vi "参数设置对话框.vi"() -> ()   [LabVIEW 2016, in "科盛超标留样.lvlib"]
uses:
  <vilib>/Utility/config.llb/NI_LVConfig.lvlib
panel:
  out "表格控件":string[][](table)
  out "查询采样记录":T1(array[cluster])
  out "查询瓶记录":T2
  in  "关闭":bool
  in  "清除瓶记录":bool
  in  "切换串口":bool
  in  "查询瓶记录":bool
  in  "查询采样记录":bool
  in  "VISA resource name":refnum<visa-resource-name>="COM10" caption="VISA资源名称"
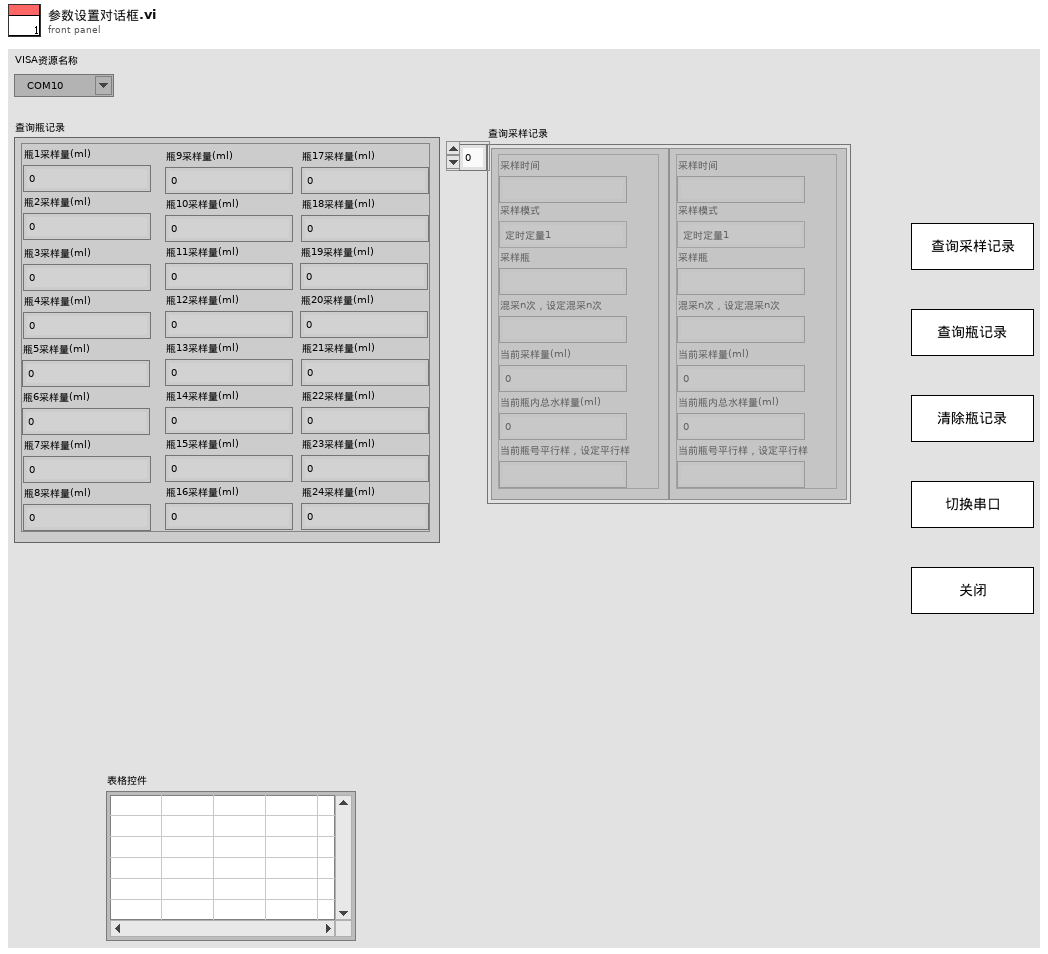
[diagram p1: front panel]
types:
  T1 = cluster{"采样时间":string, "采样模式":enum16{"定时定量1", "定时定量2", "定流定量", "定时比例", "同步留样", "超标留样", "触发采样", "定时采样1", "定流供样", "定时采样2", "远程取样", "手动取样", "流量跟踪"}, "采样瓶":string, "混采n次，设定混采n次":string, "当前采样量(ml)":dbl, "当前瓶内总水样量(ml)":dbl, "当前瓶号平行样，设定平行样":string}[]
  T2 = cluster{"瓶1采样量(ml)":dbl, "瓶2采样量(ml)":dbl, "瓶3采样量(ml)":dbl, "瓶4采样量(ml)":dbl, "瓶5采样量(ml)":dbl, "瓶6采样量(ml)":dbl, "瓶7采样量(ml)":dbl, "瓶8采样量(ml)":dbl, "瓶9采样量(ml)":dbl, "瓶10采样量(ml)":dbl, "瓶11采样量(ml)":dbl, "瓶12采样量(ml)":dbl, "瓶13采样量(ml)":dbl, "瓶14采样量(ml)":dbl, "瓶15采样量(ml)":dbl, "瓶16采样量(ml)":dbl, "瓶17采样量(ml)":dbl, "瓶18采样量(ml)":dbl, "瓶19采样量(ml)":dbl, "瓶20采样量(ml)":dbl, "瓶21采样量(ml)":dbl, "瓶22采样量(ml)":dbl, "瓶23采样量(ml)":dbl, "瓶24采样量(ml)":dbl}
  T3 = cluster{"枚举":enum16{"open", "read", "write", "close"}, "写入字符串":string, "解析字符串":string}
  T4 = typedef "NI_LVConfig.lvlib/Config Data RefNum.ctl" = refnum<k1>
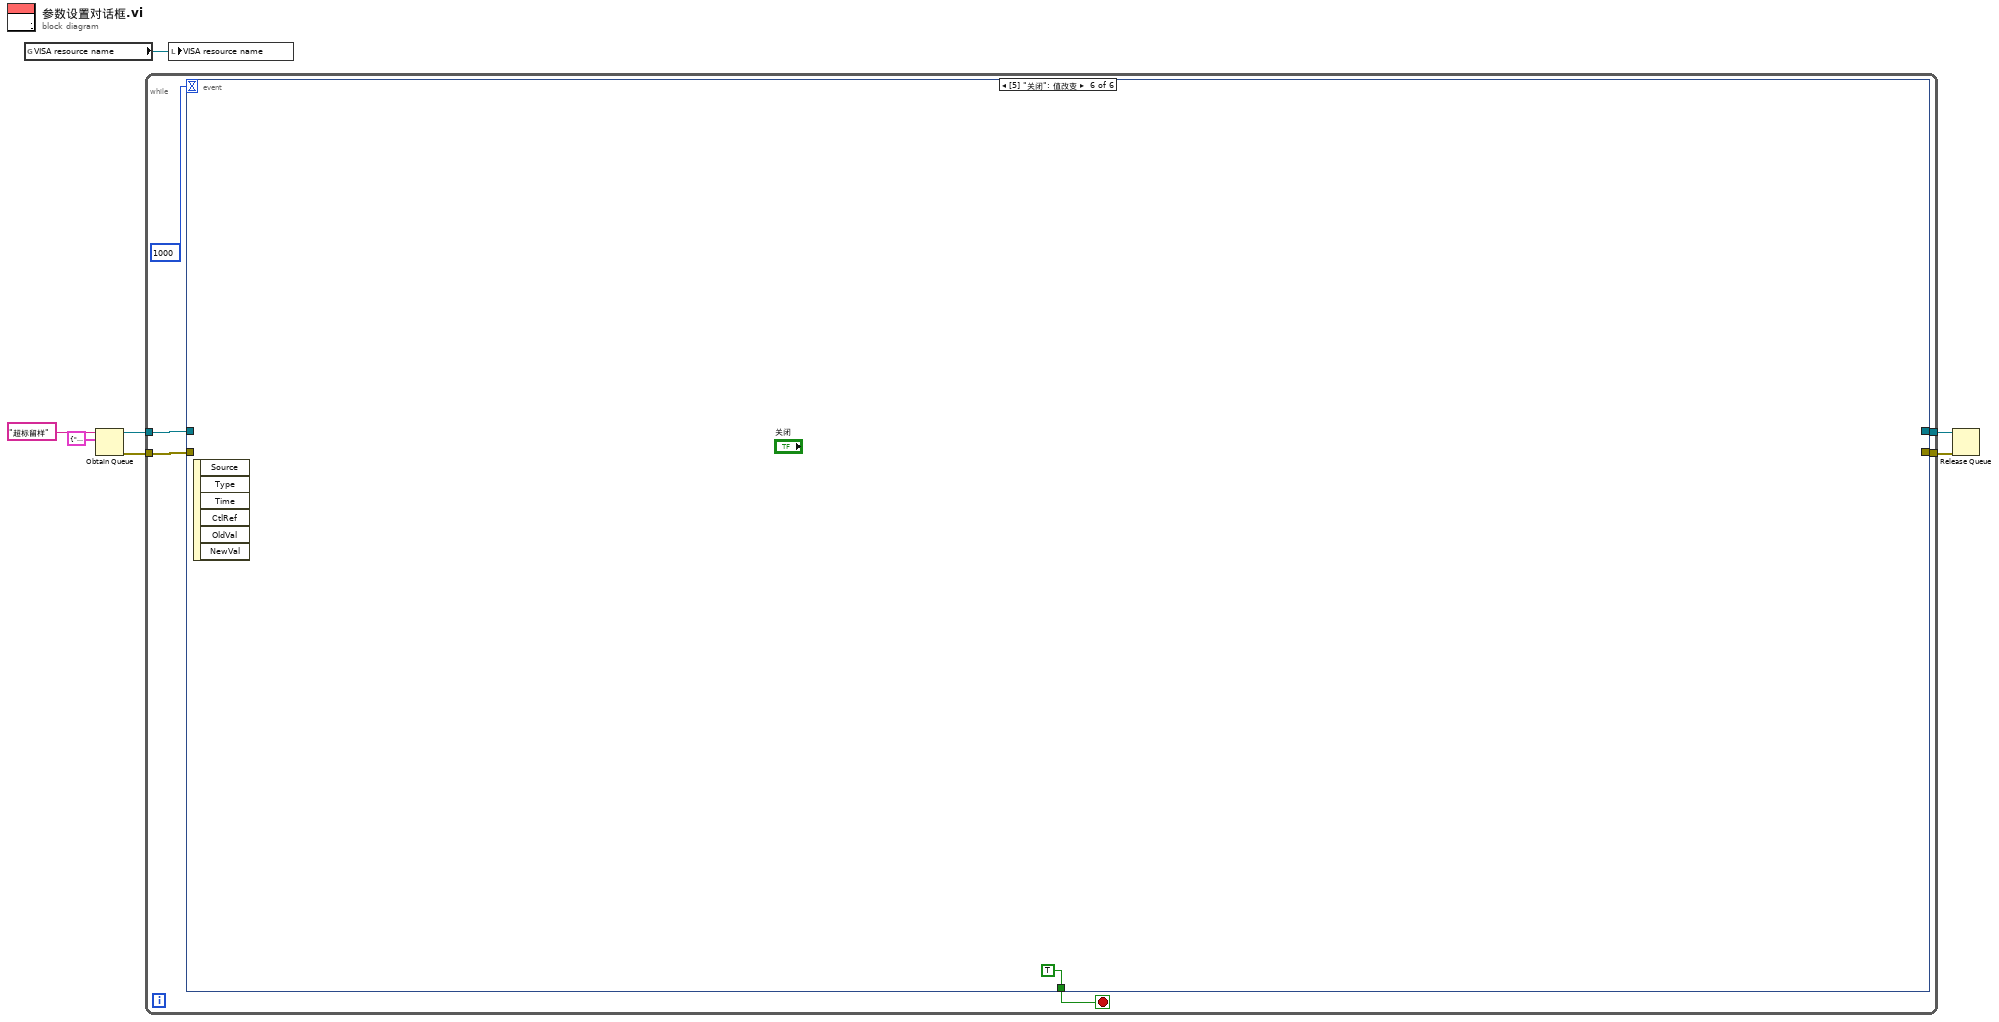
[diagram p0: block diagram]
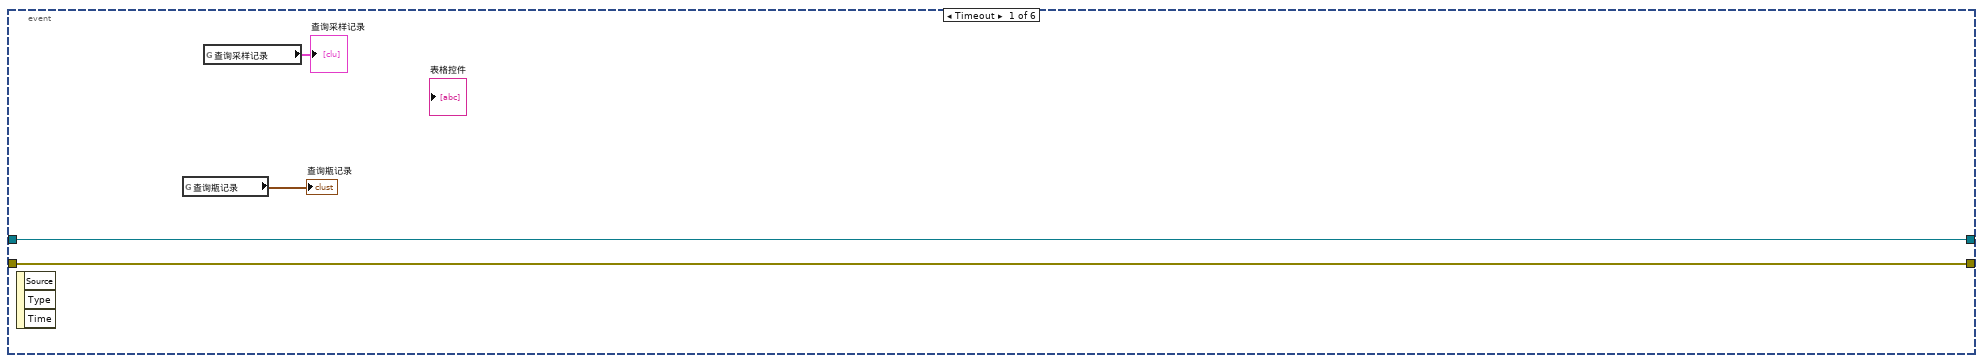
[diagram p2: hidden frame]
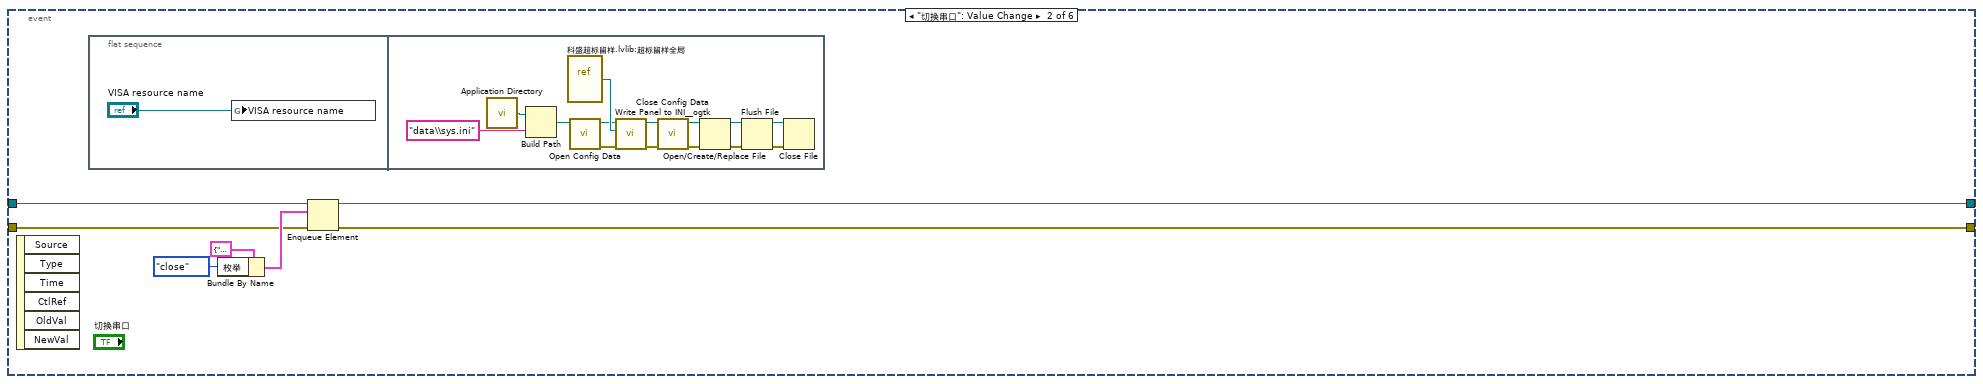
[diagram p3: hidden frame]
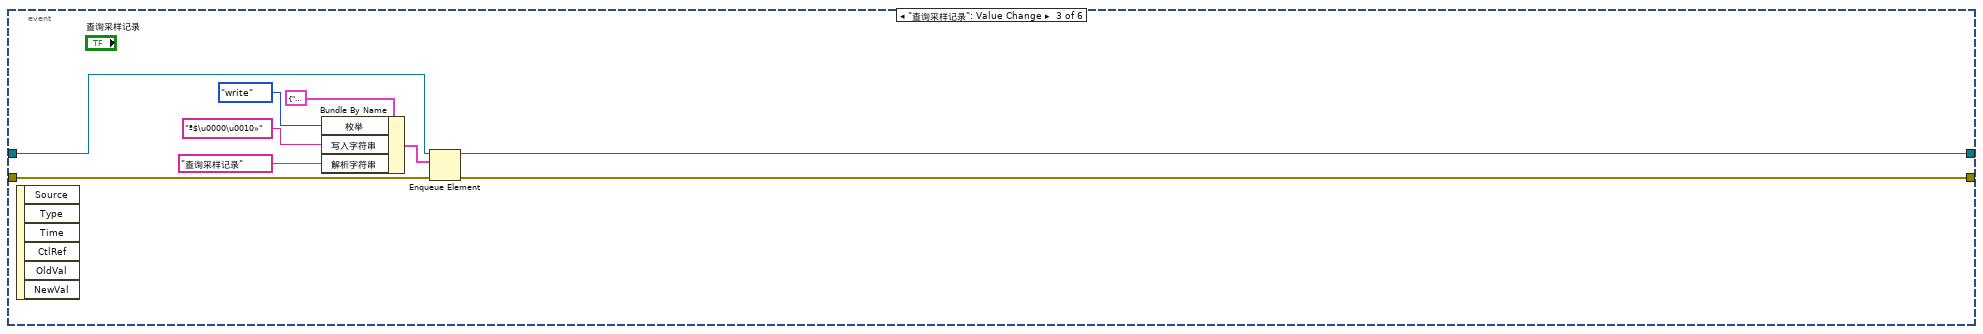
[diagram p4: hidden frame]
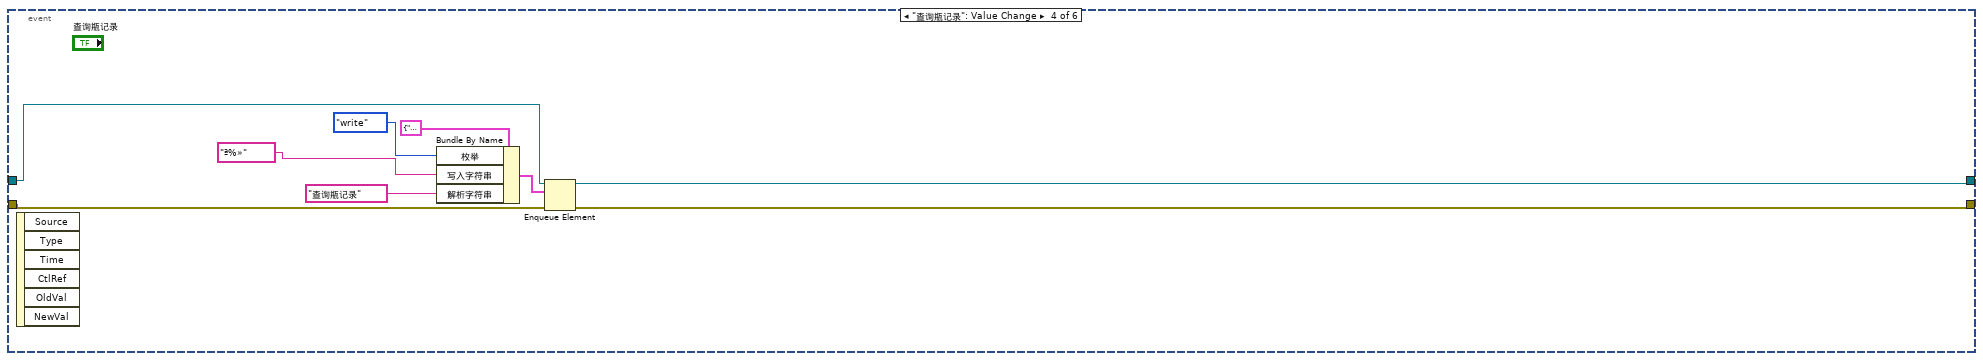
[diagram p5: hidden frame]
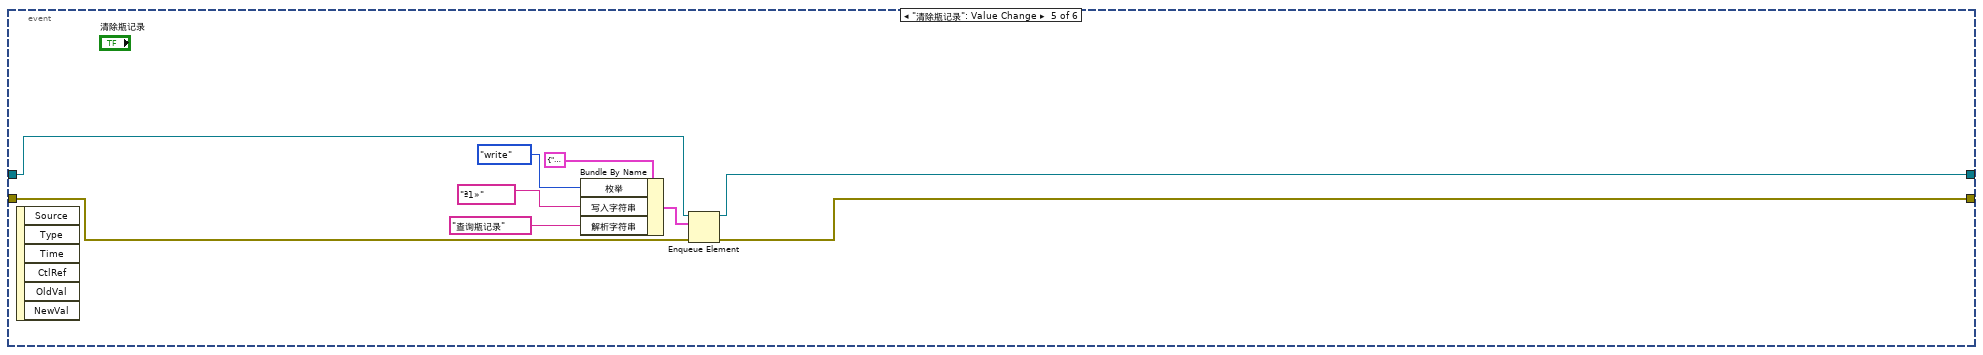
[diagram p6: hidden frame]
diagram:
  n1 = global read "超标留样全局.vi" "VISA resource name"() -> (w3:refnum<visa-resource-name>)
  n2 = Obtain Queue(name (unnamed)="超标留样" ("名称（未命名）"), element data type=T3 {"枚举"=enum."open", "写入字符串"="", "解析字符串"=""}) -> (queue out=w5:refnum<queue>, error out=w4:errorcluster)  [unwired: 3 in, 1 out]
  n3 = while {
    tunnel: w5 -> [w12]
    tunnel: w4 -> [w11]
    tunnel: [w13] -> w2
    tunnel: [w10] -> w1
    stop <- w8 stop-if-true
    n4 = event shown="[5] \"关闭\": 值改变" {
      selector: _ -> [_ _ _ _ _ _]
      dyn-events: _ -> [_ _ _ _ _ _]
      timeout: 1000 -> [_ _ _ _ _ _]
      tunnel: [w17 w19 w41 w50 w60 _] -> w13
      tunnel: w12 -> [w17 w21 w43 w53 w62 _]
      tunnel: w11 -> [w16 w20 w42 w52 w61 _]
      tunnel: [w16 w18 w40 w49 w59 _] -> w10
      tunnel: [_ _ _ _ _ TRUE] -> w8
      event Timeout {
        n5 = event-data() -> ()  [unwired: 1 in, 3 out]
        n6 = global read "超标留样全局.vi" "查询瓶记录"() -> (→"查询瓶记录":T2)
        n7 = global read "超标留样全局.vi" "查询采样记录"() -> (→"查询采样记录":T1)
      }
      event "切换串口": Value Change {
        n8 = event-data() -> ()  [unwired: 1 in, 6 out]
        n9 = flat-sequence {
          frame #0 {
            n10 = global write "超标留样全局.vi" "VISA resource name"("VISA resource name") -> ()
          }
          frame #1 {
            n11 = call <vilib>:"Application Directory.vi"() -> ("Application Directory"=w27:path)
            n12 = Build Path(base path=w27, name or relative path="data\\sys.ini" ("名称或相对路径")) -> (appended path=w28:path)
            n13 = vi-ref "科盛超标留样.lvlib:超标留样全局.vi"() -> (w30:refnum<vi>)
            n14 = call <vilib>:"Open Config Data.vi"("configuration file path"=w28) -> ("error out"=w32:errorcluster, "refnum"=w29:T4)  [unwired: 8 in, 1 out]
            n15 = call <userlib>:"Write Panel to INI__ogtk.vi"("error in (no error)"=w32, "VI ref"=w30, "refnum"=w29) -> ("error out"=w33:errorcluster, "refnum out"=w31:T4)  [unwired: 7 in]
            n16 = call <vilib>:"Close Config Data.vi"("error in (no error)"=w33, "refnum"=w31) -> ("error out"=w38:errorcluster, "file path"=w39:path)  [unwired: 8 in]
            n17 = Open/Create/Replace File(file path (use dialog)=w39, error in=w38) -> (refnum out=w35:refnum<file>, error out=w34:errorcluster)  [unwired: 4 in, 1 out]
            n18 = Flush File(refnum=w35, error in=w34) -> (refnum out=w36:refnum<file>, error out=w37:errorcluster)
            n19 = Close File(refnum=w36, error in=w37) -> ()  [unwired: 2 out]
          }
        }
        n20 = Bundle By Name(cluster=T3 {"枚举"=enum."open", "写入字符串"="", "解析字符串"=""}, "枚举"=enum16{"open", "read", "write", "close"}."close" ("元素")) -> (w23:T3)
        n21 = Enqueue Element(queue=w21, element=w23, error in (no error)=w20) -> (queue out=w19:refnum<queue>, error out=w18:errorcluster)  [unwired: 1 in, 1 out]
      }
      event "查询采样记录": Value Change {
        n22 = event-data() -> ()  [unwired: 1 in, 6 out]
        n23 = Bundle By Name(cluster=T3 {"枚举"=enum."open", "写入字符串"="", "解析字符串"=""}, "枚举"=enum16{"open", "read", "write", "close"}."write" ("元素"), "写入字符串"="ª$\u0000\u0010»" ("写入缓冲区"), "解析字符串"="查询采样记录" ("当前解析模式")) -> (w44:T3)
        n24 = Enqueue Element(queue=w43, element=w44, error in (no error)=w42) -> (queue out=w41:refnum<queue>, error out=w40:errorcluster)  [unwired: 1 in, 1 out]
      }
      event "查询瓶记录": Value Change {
        n25 = event-data() -> ()  [unwired: 1 in, 6 out]
        n26 = Bundle By Name(cluster=T3 {"枚举"=enum."open", "写入字符串"="", "解析字符串"=""}, "枚举"=enum16{"open", "read", "write", "close"}."write" ("元素"), "写入字符串"="ª%»" ("写入缓冲区"), "解析字符串"="查询瓶记录" ("当前解析模式")) -> (w54:T3)
        n27 = Enqueue Element(queue=w53, element=w54, error in (no error)=w52) -> (queue out=w50:refnum<queue>, error out=w49:errorcluster)  [unwired: 1 in, 1 out]
      }
      event "清除瓶记录": Value Change {
        n28 = event-data() -> ()  [unwired: 1 in, 6 out]
        n29 = Bundle By Name(cluster=T3 {"枚举"=enum."open", "写入字符串"="", "解析字符串"=""}, "枚举"=enum16{"open", "read", "write", "close"}."write" ("元素"), "写入字符串"="ª1»" ("写入缓冲区"), "解析字符串"="查询瓶记录" ("当前解析模式")) -> (w63:T3)
        n30 = Enqueue Element(queue=w62, element=w63, error in (no error)=w61) -> (queue out=w60:refnum<queue>, error out=w59:errorcluster)  [unwired: 1 in, 1 out]
      }
      event "关闭": Value Change {
        n31 = event-data() -> ()  [unwired: 1 in, 6 out]
      }
    }
  }
  n32 = local write "VISA resource name"(w3) -> ()
  n33 = Release Queue(queue=w2, error in (no error)=w1) -> ()  [unwired: 1 in, 3 out]
